vi "strings to base format.vi"(8 "error in":errorcluster, 11 "1.0.0":T1) -> (0 "error out":errorcluster, 3 "format":T4)   [LabVIEW 2013, in "NISE_CEF_TreeSerializer.lvlib"]
uses:
  NISE_CEF_TreeSerializer.lvlib
  base file format.ctl
  file data format.ctl
  hierarchy element.ctl
  instance data.ctl
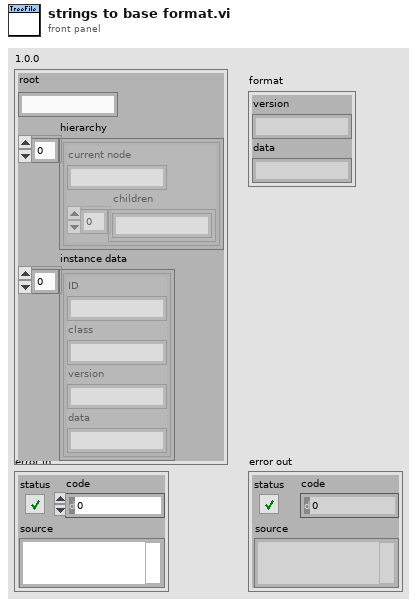
[diagram p1: front panel]
types:
  T1 = typedef "NISE_CEF_TreeSerializer.lvlib/file data format.ctl" = cluster{"root":string, "hierarchy":T2[], "instance data":T3[]}
  T2 = typedef "NISE_CEF_TreeSerializer.lvlib/hierarchy element.ctl" = cluster{"current node":string, "children":string[]}
  T3 = typedef "NISE_CEF_TreeSerializer.lvlib/instance data.ctl" = cluster{"ID":string, "class":string, "version":string, "data":string}
  T4 = typedef "NISE_CEF_TreeSerializer.lvlib/base file format.ctl" = cluster{"version":string, "data":string}
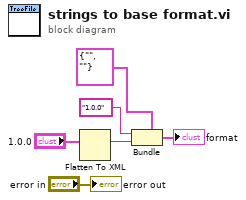
[diagram p0: block diagram]
diagram:
  n1 = Flatten To XML(anything="1.0.0") -> (xml string=w2:string)
  n2 = Bundle(cluster=T4 {"version"="", "data"=""} ("format"), "version"="1.0.0", "data"=w2) -> (→"format":T4)
  "error out" <- "error in"
